vi "Get Property.vi"(0 "SLSC Remote in":refnum<class "SLSC Remote.lvclass">, 1 "property type":T1, 5 "property":refnum<k21>, 7 "resources":string, 11 "error in (no error)":errorcluster) -> (4 "SLSC Remote out":refnum<class "SLSC Remote.lvclass">, 10 "property value":variant, 15 "error out":errorcluster)   [LabVIEW 2015, in "SLSC Remote.lvclass"]
uses:
  SLSC Remote.lvclass
  SLSC Interface Class/Property Type.ctl
  <vilib>/NI/i3 JSON/JSON Generation/Create Value Files/Create Value - Object.vi
  <vilib>/NI/i3 JSON/JSON Generation/Add Object Parameter Files/Add Object Parameter - String.vi
  <vilib>/NI/NI JSONRPC Server Framework/Classes/Server/Format Client Request (Auto-Increment).vi
  <vilib>/httpClient/POSTBuffer.vi
  <vilib>/NI/i3 JSON/JSON Parsing/Get Object Parameter Files/Get Object Parameter - Boolean.vi
  <vilib>/NI/i3 JSON/JSON Parsing/Get Object Parameter Files/Get Object Parameter - Numeric.vi
  <vilib>/NI/i3 JSON/JSON Parsing/Get Object Parameter Files/Get Object Parameter - String.vi
  <vilib>/NI/i3 JSON/JSON Parsing/Get Object Parameter Files/Get Object Parameter - 1D Array Boolean.vi
  <vilib>/NI/i3 JSON/JSON Parsing/Get Object Parameter Files/Get Object Parameter - 1D Array Double.vi
  <vilib>/NI/i3 JSON/JSON Parsing/Get Object Parameter Files/Get Object Parameter - 1D Array String.vi
  <vilib>/NI/NI JSONRPC Server Framework/Classes/Server/JSONRPC Server.lvclass
  <vilib>/NI/i3 JSON/i3-json.lvlib
  <vilib>/httpClient/LabVIEWHTTPClient.lvlib
  SLSC Interface Class/SLSC Interface.lvclass
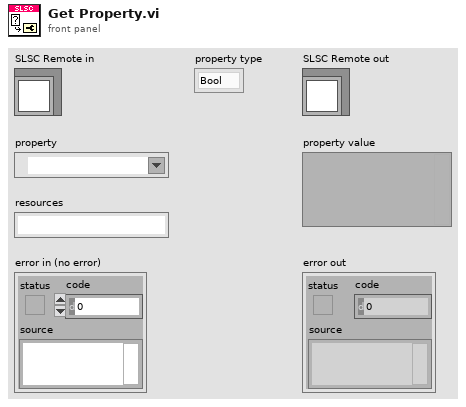
[diagram p1: front panel]
types:
  T1 = typedef "SLSC Interface.lvclass/Property Type.ctl" = enum16{"Bool", "DBL", "I32", "I64", "String", "U32", "U64", "1D Bool", "1D DBL", "1D I32", "1D I64", "1D String", "1D U32", "1D U64"}
  T2 = typedef "LabVIEWHTTPClient.lvlib/ClientHandle.ctl" = refnum<k1>
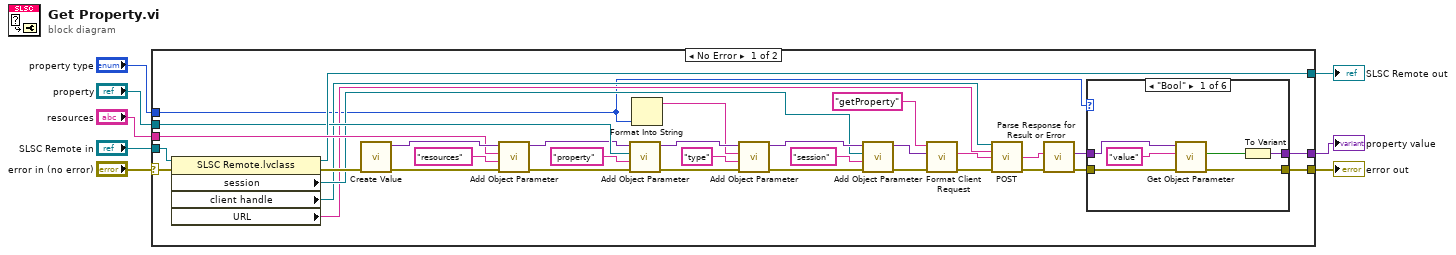
[diagram p0: block diagram]
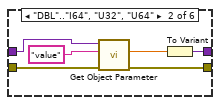
[diagram p2: hidden frame]
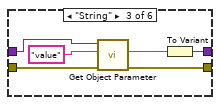
[diagram p3: hidden frame]
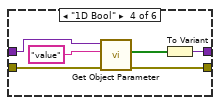
[diagram p4: hidden frame]
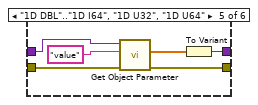
[diagram p5: hidden frame]
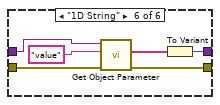
[diagram p6: hidden frame]
diagram:
  n1 = case shown="No Error" "error in (no error)" {
    selector: "error in (no error)" -> [w35 w79]
    tunnel: "resources" -> [w41 _]
    tunnel: "SLSC Remote in" -> [w39 w80]
    tunnel: [w38 w80] -> w3
    tunnel: "property" -> [w36 _]
    tunnel: "property type" -> [w13 _]
    tunnel: [w10 w79] -> w2
    tunnel: [w9 _] -> w1
    frame No Error {
      n2 = property class="SLSC Remote.lvclass"(reference=w39, error in=w35) -> (reference out=w38:refnum<class "SLSC Remote.lvclass">, error out=w34:errorcluster, "session"=w24:refnum<k21>, "client handle"=w20:T2, "URL"=w19:string)
      n3 = call-poly <vilib>:"Create Value.vi"("error in (no error)"=w34) -> ("error out"=w33:errorcluster, "JSON Tree"=w42:variant)  [unwired: 9 in]
      n4 = call-poly <vilib>:"Add Object Parameter.vi"("error in (no error)"=w33, "Name"="resources", "String"=w41, "JSON Tree in (JSON Object)"=w42) -> ("error out"=w32:errorcluster, "JSON Tree out (JSON Object)"=w29:variant)  [unwired: 6 in]
      n5 = call-poly <vilib>:"Add Object Parameter.vi"("error in (no error)"=w32, "Name"="property", "String"=w36, "JSON Tree in (JSON Object)"=w29) -> ("error out"=w27:errorcluster, "JSON Tree out (JSON Object)"=w28:variant)  [unwired: 6 in]
      n6 = Format Into String(w13) -> (resulting string=w16:string)  [unwired: 3 in, 1 out]
      n7 = call-poly <vilib>:"Add Object Parameter.vi"("error in (no error)"=w27, "Name"="type" ("String"), "String"=w16, "JSON Tree in (JSON Object)"=w28) -> ("error out"=w25:errorcluster, "JSON Tree out (JSON Object)"=w26:variant)  [unwired: 6 in]
      n8 = call-poly <vilib>:"Add Object Parameter.vi"("error in (no error)"=w25, "Name"="session", "String"=w24, "JSON Tree in (JSON Object)"=w26) -> ("error out"=w21:errorcluster, "JSON Tree out (JSON Object)"=w22:variant)  [unwired: 6 in]
      n9 = call-poly <vilib>:"Format Client Request.vi"("error in (no error)"=w21, "params"=w22, "method"="getProperty") -> ("error out"=w18:errorcluster, "Request String"=w30:string)  [unwired: 7 in]
      n10 = call-poly <vilib>:"POST.vi"("client handle"=w20, "url"=w19, "buffer"=w30, "error in (no error)"=w18) -> ("body"=w15:string, "error out"=w14:errorcluster)  [unwired: 8 in, 2 out]
      n11 = call <vilib>:"Parse Response for Result or Error.vi"("error in"=w14, "Response String In"=w15) -> ("error out"=w11:errorcluster, "Result or Error Data"=w12:variant)  [unwired: 7 in, 1 out]
      n12 = case shown="\"Bool\"" w13 {
        tunnel: w12 -> [w48 w54 w60 w66 w72 w78]
        tunnel: w11 -> [w46 w52 w58 w64 w70 w76]
        tunnel: [w45 w51 w57 w63 w69 w75] -> w10
        tunnel: [w43 w49 w55 w61 w67 w73] -> w9
        frame "Bool" {
          n13 = call-poly <vilib>:"Get Object Parameter.vi"("error in (no error)"=w46, "Parameter Name"="value", "JSON Tree In (JSON Object)"=w48) -> ("error out"=w45:errorcluster, "Boolean Value"=w44:bool)  [unwired: 5 in, 2 out]
          n14 = To Variant(anything=w44) -> (Variant=w43:variant)
        }
        frame "DBL".."I64", "U32", "U64" {
          n15 = call-poly <vilib>:"Get Object Parameter.vi"("error in (no error)"=w52, "Parameter Name"="value", "JSON Tree In (JSON Object)"=w54) -> ("error out"=w51:errorcluster, "Double Value"=w50:dbl)  [unwired: 5 in, 2 out]
          n16 = To Variant(anything=w50) -> (Variant=w49:variant)
        }
        frame "String" {
          n17 = call-poly <vilib>:"Get Object Parameter.vi"("error in (no error)"=w58, "Parameter Name"="value", "JSON Tree In (JSON Object)"=w60) -> ("error out"=w57:errorcluster, "String Value"=w56:string)  [unwired: 5 in, 2 out]
          n18 = To Variant(anything=w56) -> (Variant=w55:variant)
        }
        frame "1D Bool" {
          n19 = call-poly <vilib>:"Get Object Parameter.vi"("error in (no error)"=w64, "Parameter Name"="value", "JSON Tree In (JSON Object)"=w66) -> ("error out"=w63:errorcluster, "1D Boolean Array Value"=w62:bool[])  [unwired: 5 in, 2 out]
          n20 = To Variant(anything=w62) -> (Variant=w61:variant)
        }
        frame "1D DBL".."1D I64", "1D U32", "1D U64" {
          n21 = call-poly <vilib>:"Get Object Parameter.vi"("error in (no error)"=w70, "Parameter Name"="value", "JSON Tree In (JSON Object)"=w72) -> ("error out"=w69:errorcluster, "1D Double Array Value"=w68:dbl[])  [unwired: 5 in, 2 out]
          n22 = To Variant(anything=w68) -> (Variant=w67:variant)
        }
        frame "1D String" {
          n23 = call-poly <vilib>:"Get Object Parameter.vi"("error in (no error)"=w76, "Parameter Name"="value", "JSON Tree In (JSON Object)"=w78) -> ("error out"=w75:errorcluster, "1D String Array Value"=w74:string[])  [unwired: 5 in, 2 out]
          n24 = To Variant(anything=w74) -> (Variant=w73:variant)
        }
      }
    }
    frame Error {
    }
  }
  "error out" <- w2
  "SLSC Remote out" <- w3
  "property value" <- w1
